vi "Others.vi"() -> ()   [LabVIEW 2019]
uses:
  <vilib>/numeric/Random Number (Range) U64.vi
  <vilib>/numeric/sub_Random U32.vi
panel:
  out "s? t:f":string
  in  "False Statement":string
  in  "True Statement":string
  out "number":u64
  in  "lower bound (0)":u64
  in  "upper bound (1000)":u64=100
  in  "y":dbl
  in  "x":dbl
  in  "s":bool
  out "min(x,y)":dbl
  out "max(x,y)":dbl
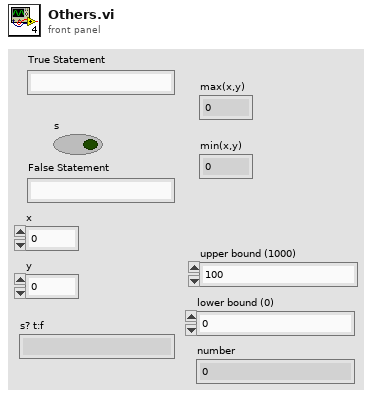
[diagram p1: front panel]
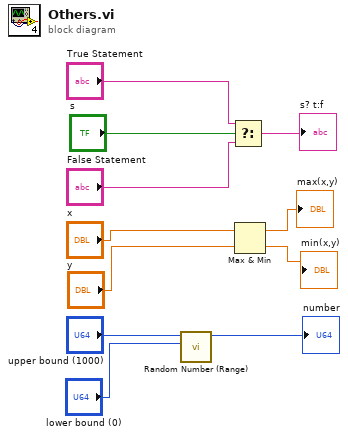
[diagram p0: block diagram]
diagram:
  n1 = call-poly <vilib>:"Random Number (Range).vi"("lower bound (0)"="lower bound (0)", "upper bound (100)"="upper bound (1000)") -> ("number"=→"number":u64)  [unwired: 9 in]
  n2 = Select(t="True Statement", s="s", f="False Statement") -> (s? t:f=→"s? t:f":string)
  n3 = Max & Min(x="x", y="y") -> (max(x,y)=→"max(x,y)":dbl, min(x,y)=→"min(x,y)":dbl)
